vi "NI-9205_SoftPanel.vi"(3 "NI-9205 in Slot:":string="1") -> ()   [LabVIEW 2016]
uses:
  GlobalControlVariables.vi
panel:
  in  "AI 15 Level":string(combo)="0.2V"
  in  "AI 14 Level":string(combo)="0.2V"
  in  "AI 13 Level":string(combo)="0.2V"
  in  "AI 12 Level":string(combo)="0.2V"
  in  "AI 11 Level":string(combo)="0.2V"
  in  "AI 10 Level":string(combo)="0.2V"
  in  "AI 09 Level":string(combo)="0.2V"
  in  "AI 08 Level":string(combo)="0.2V"
  in  "AI 07 Level":string(combo)="0.2V"
  in  "AI 06 Level":string(combo)="0.2V"
  in  "AI 05 Level":string(combo)="0.2V"
  in  "AI 04 Level":string(combo)="0.2V"
  in  "AI 03 Level":string(combo)="0.2V"
  in  "AI 02 Level":string(combo)="0.2V"
  in  "AI 01 Level":string(combo)="0.2V"
  in  "AI 00 Level":string(combo)="0.2V"
  in  "AI 06 & 14 Select":string(combo)="S"
  in  "AI 07 & 15 Select":string(combo)="S"
  in  "AI 05 & 13 Select":string(combo)="S"
  in  "AI 02 & 10 Select":string(combo)="S"
  in  "AI 04 & 12 Select":string(combo)="S"
  in  "AI 03 & 11 Select":string(combo)="S"
  in  "AI 01 & 09 Select":string(combo)="S"
  out "AI Values":dbl[](array[numeric])
  out "ExitModule":bool=TRUE
  out "AI 07":dbl
  out "AI 06":dbl
  out "AI 05":dbl
  out "AI 04":dbl
  out "AI 03":dbl
  out "AI 02":dbl
  out "AI 01":dbl
  out "AI 00":dbl
  out "AI 15":dbl min=0.0 max=5.0
  out "AI 14":dbl min=0.0 max=5.0
  out "AI 13":dbl min=0.0 max=5.0
  out "AI 12":dbl min=0.0 max=5.0
  out "AI 11":dbl min=0.0 max=5.0
  out "AI 10":dbl min=0.0 max=5.0
  out "AI 09":dbl min=0.0 max=5.0
  out "AI 08":dbl min=0.0 max=5.0
  in  "Submit Levels":bool
  in  "Submit Differentials":bool
  in  "AI 00 & 08 Select":string(combo)="S"
  in  "ExitButton":bool
  # "Analog Levels"
  # "Analog Inputs"
  # "Analog Differential Pairs"
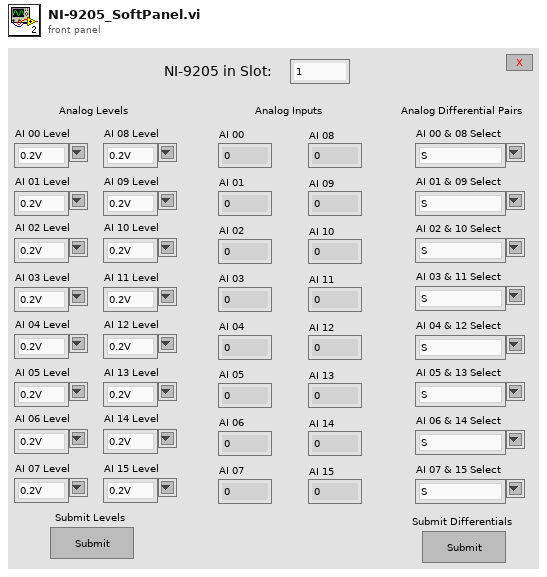
[diagram p1: front panel]
types:
  T1 = cluster{"AI Values[0]":dbl, "AI Values[1]":dbl, "AI Values[2]":dbl, "AI Values[3]":dbl, "AI Values[4]":dbl, "AI Values[5]":dbl, "AI Values[6]":dbl, "AI Values[7]":dbl, "AI Values[8]":dbl, "AI Values[9]":dbl, "AI Values[10]":dbl, "AI Values[11]":dbl, "AI Values[12]":dbl, "AI Values[13]":dbl, "AI Values[14]":dbl, "AI Values[15]":dbl}
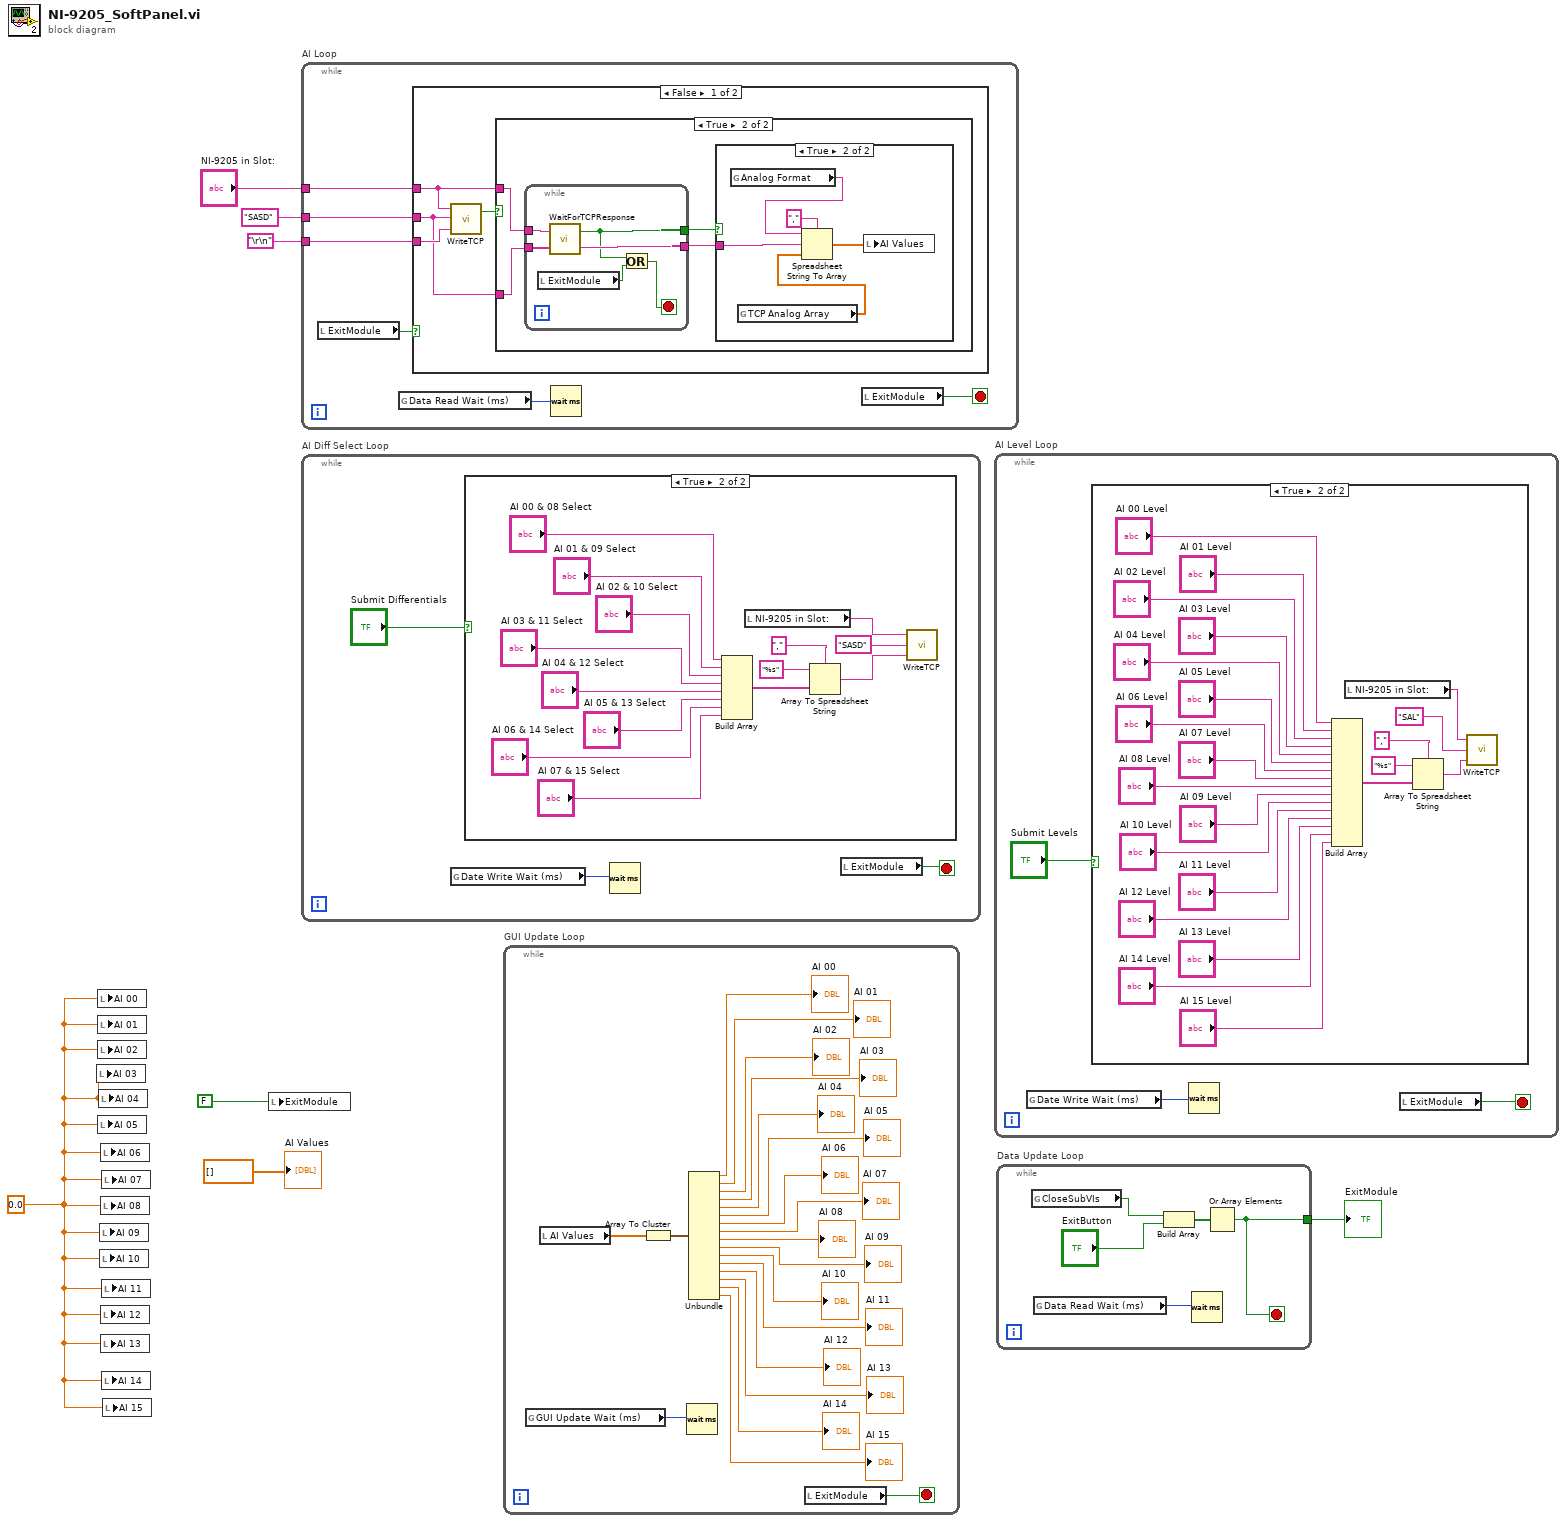
[diagram p0: block diagram]
diagram:
  w4 = 0.0
  n1 = local write "AI 03"(w4) -> ()
  n2 = local write "AI 00"(w4) -> ()
  n3 = local write "AI 01"(w4) -> ()
  n4 = local write "AI 02"(w4) -> ()
  n5 = local write "AI 05"(w4) -> ()
  n6 = local write "AI 04"(w4) -> ()
  n7 = local write "AI 09"(w4) -> ()
  n8 = local write "AI 10"(w4) -> ()
  n9 = local write "AI 06"(w4) -> ()
  n10 = local write "AI 08"(w4) -> ()
  n11 = local write "AI 12"(w4) -> ()
  n12 = local write "AI 13"(w4) -> ()
  n13 = local write "AI 07"(w4) -> ()
  n14 = local write "AI 11"(w4) -> ()
  n15 = local write "AI 14"(w4) -> ()
  n16 = local write "AI 15"(w4) -> ()
  n17 = local write "ExitModule"(FALSE) -> ()
  n18 = while "AI Loop" {
    tunnel: "NI-9205 in Slot:" -> [w12]
    tunnel: "\r\n" -> [w10]
    tunnel: "SASD" -> [w9]
    stop <- w13 stop-if-true
    n19 = local read "ExitModule"() -> (w8:bool)
    n20 = global read "GlobalControlVariables.vi" "Data Read Wait (ms)"() -> (w11:u32)
    n21 = case shown="False" w8 {
      tunnel: w12 -> [w16 _]
      tunnel: w10 -> [w15 _]
      tunnel: w9 -> [w14 _]
      frame False {
        n22 = call "WriteTCP.vi"("Data"=w15, "Action"=w14, "Module Slot"=w16) -> ("Sent"=w17:bool)  [unwired: 1 out]
        n23 = case shown="True" w17 {
          tunnel: w16 -> [_ w20]
          tunnel: w14 -> [_ w19]
          frame False {
          }
          frame True {
            n24 = while {
              tunnel: [w22] -> w21
              tunnel: w20 -> [w27]
              tunnel: w19 -> [w26]
              tunnel: [w25] -> w18
              stop <- w23 stop-if-true
              n25 = local read "ExitModule"() -> (w24:bool)
              n26 = call "WaitForTCPResponse.vi"("Action"=w26, "Module Slot"=w27) -> ("Received Data"=w25:string, "Ready"=w22:bool)
              n27 = Or(x=w22, y=w24) -> (x .or. y?=w23:bool)
            }
            n28 = case shown="True" w21 {
              tunnel: w18 -> [_ w32]
              frame False {
              }
              frame True {
                n29 = global read "GlobalControlVariables.vi" "Analog Format"() -> (w29:string)
                n30 = global read "GlobalControlVariables.vi" "TCP Analog Array"() -> (w30:dbl[])
                n31 = Spreadsheet String To Array(delimiter (Tab)=",", format string=w29, spreadsheet string=w32, array type (2D Dbl)=w30) -> (array=w28:dbl[])
                n32 = local write "AI Values"(w28) -> ()
              }
            }
          }
        }
      }
      frame True {
      }
    }
    n33 = Wait (ms)(milliseconds to wait=w11) -> ()  [unwired: 1 out]
    n34 = local read "ExitModule"() -> (w13:bool)
  }
  n35 = while "AI Diff Select Loop" {
    stop <- w33 stop-if-true
    n36 = global read "GlobalControlVariables.vi" "Date Write Wait (ms)"() -> (w34:u32)
    n37 = case shown="True" "Submit Differentials" {
      frame False {
      }
      frame True {
        n38 = Build Array("AI 00 & 08 Select", "AI 01 & 09 Select", "AI 02 & 10 Select", "AI 03 & 11 Select", "AI 04 & 12 Select", "AI 05 & 13 Select", "AI 06 & 14 Select", "AI 07 & 15 Select") -> (w44:string[])
        n39 = local read "NI-9205 in Slot:"() -> (w48:string)
        n40 = Array To Spreadsheet String(delimiter (Tab)=",", array=w44, 3:"%s") -> (spreadsheet string=w47:string)
        n41 = call "WriteTCP.vi"("Data"=w47, "Action"="SASD", "Module Slot"=w48) -> ()  [unwired: 2 out]
      }
    }
    n42 = Wait (ms)(milliseconds to wait=w34) -> ()  [unwired: 1 out]
    n43 = local read "ExitModule"() -> (w33:bool)
  }
  n44 = while "GUI Update Loop" {
    stop <- w58 stop-if-true
    n45 = global read "GlobalControlVariables.vi" "GUI Update Wait (ms)"() -> (w69:u32)
    n46 = local read "AI Values"() -> (w59:dbl[])
    n47 = Array To Cluster(array=w59) -> (cluster=w68:T1)
    n48 = Wait (ms)(milliseconds to wait=w69) -> ()  [unwired: 1 out]
    n49 = Unbundle(w68) -> ("AI Values[0]"=→"AI 00":dbl, "AI Values[1]"=→"AI 01":dbl, "AI Values[2]"=→"AI 02":dbl, "AI Values[3]"=→"AI 03":dbl, "AI Values[4]"=→"AI 04":dbl, "AI Values[5]"=→"AI 05":dbl, "AI Values[6]"=→"AI 06":dbl, "AI Values[7]"=→"AI 07":dbl, "AI Values[8]"=→"AI 08":dbl, "AI Values[9]"=→"AI 09":dbl, "AI Values[10]"=→"AI 10":dbl, "AI Values[11]"=→"AI 11":dbl, "AI Values[12]"=→"AI 12":dbl, "AI Values[13]"=→"AI 13":dbl, "AI Values[14]"=→"AI 14":dbl, "AI Values[15]"=→"AI 15":dbl)
    n50 = local read "ExitModule"() -> (w58:bool)
  }
  n51 = while "AI Level Loop" {
    stop <- w71 stop-if-true
    n52 = global read "GlobalControlVariables.vi" "Date Write Wait (ms)"() -> (w70:u32)
    n53 = case shown="True" "Submit Levels" {
      frame False {
      }
      frame True {
        n54 = Build Array("AI 00 Level", "AI 01 Level", "AI 02 Level", "AI 03 Level", "AI 04 Level", "AI 05 Level", "AI 06 Level", "AI 07 Level", "AI 08 Level", "AI 09 Level", "AI 10 Level", "AI 11 Level", "AI 12 Level", "AI 13 Level", "AI 14 Level", "AI 15 Level") -> (w87:string[])
        n55 = local read "NI-9205 in Slot:"() -> (w90:string)
        n56 = Array To Spreadsheet String(delimiter (Tab)=",", array=w87, 3:"%s") -> (spreadsheet string=w92:string)
        n57 = call "WriteTCP.vi"("Data"=w92, "Action"="SAL", "Module Slot"=w90) -> ()  [unwired: 2 out]
      }
    }
    n58 = Wait (ms)(milliseconds to wait=w70) -> ()  [unwired: 1 out]
    n59 = local read "ExitModule"() -> (w71:bool)
  }
  n60 = while "Data Update Loop" {
    tunnel: [w95] -> w7
    stop <- w95 stop-if-true
    n61 = global read "GlobalControlVariables.vi" "CloseSubVIs"() -> (w96:bool)
    n62 = global read "GlobalControlVariables.vi" "Data Read Wait (ms)"() -> (w99:u32)
    n63 = Build Array(w96, "ExitButton") -> (w98:bool[])
    n64 = Wait (ms)(milliseconds to wait=w99) -> ()  [unwired: 1 out]
    n65 = Or Array Elements(Boolean array=w98) -> (logical OR=w95:bool)
  }
  "ExitModule" <- w7
  "AI Values" <- dbl[] []
